vi "poll.vi"(8 "error in (no error)":errorcluster, 11 "output_request_poller in":refnum<class "output_poller.lvclass">) -> (0 "error out":errorcluster, 3 "output_request_poller out":refnum<class "output_poller.lvclass">)   [LabVIEW 2015, in "output_poller.lvclass"]
uses:
  output_poller.lvclass
  output_poller.lvclass/output_poller.ctl
  <vilib>/ActorFramework/Actor/Actor.lvclass/Actor.ctl
  <vilib>/ActorFramework/Message Enqueuer/Message Enqueuer.lvclass/Message Enqueuer.ctl
  <vilib>/ActorFramework/Message Enqueuer/Init from Existing Queue.vi
  <vilib>/ActorFramework/Message Enqueuer/Enqueue.vi
  <vilib>/ActorFramework/Message Priority Queue/Priority Enqueue.vi
  <vilib>/ActorFramework/Stop Msg/Stop Msg.lvclass
  <vilib>/ActorFramework/Message Enqueuer/Message Enqueuer.lvclass
  <vilib>/ActorFramework/Actor/Actor.lvclass
  request/request.lvclass
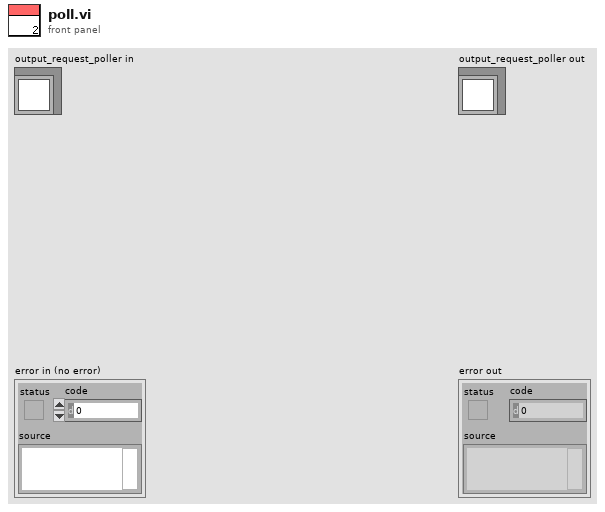
[diagram p1: front panel]
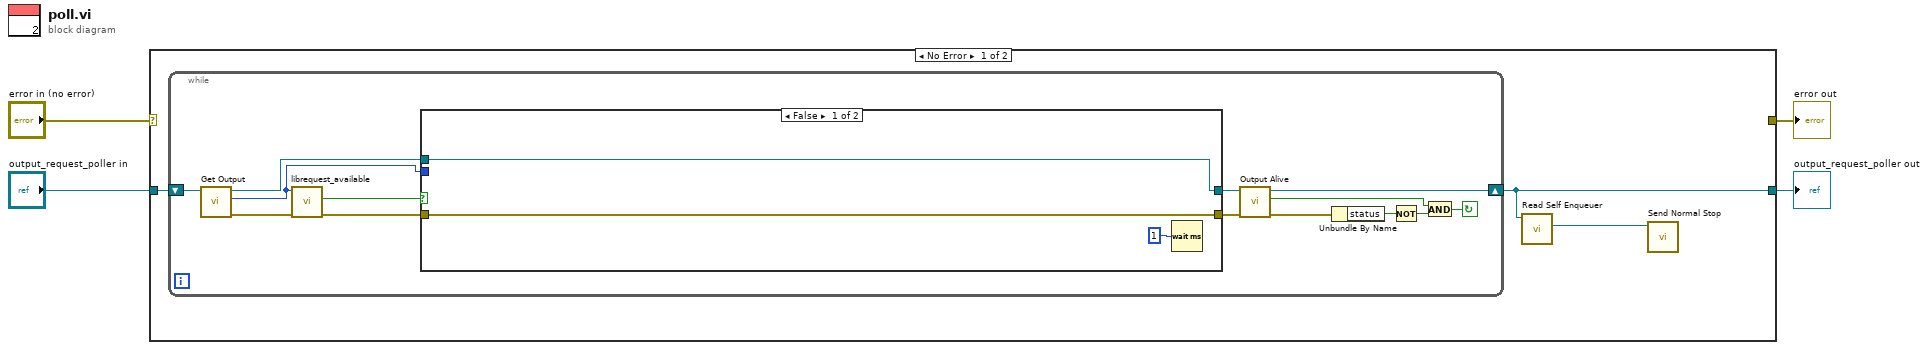
[diagram p0: block diagram]
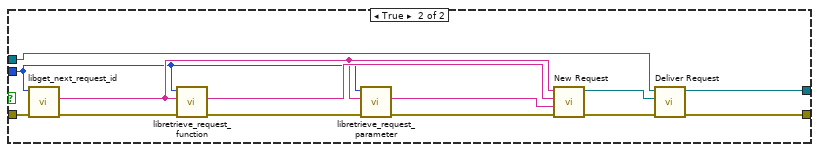
[diagram p2: hidden frame]
diagram:
  n1 = case shown="No Error" "error in (no error)" {
    selector: "error in (no error)" -> [_ w39]
    tunnel: [_ w39] -> w3
    tunnel: [w6 w38] -> w1
    tunnel: "output_request_poller in" -> [w7 w38]
    frame No Error {
      n2 = while {
        shift-right: [w20] -> w6
        shift-left: w7 -> [w17]
        stop <- w8 continue-if-true
        n3 = call "Get Output.vi"("output_request_poller in"=w17) -> ("error out"=w16:errorcluster, "output"=w14:i32, "output_request_poller out"=w15:refnum<class "output_poller.lvclass">)  [unwired: 8 in]
        n4 = call "librequest_available.vi"("error in (no error)"=w16, "output"=w14) -> ("error out"=w18:errorcluster, "is"=w19:bool)  [unwired: 8 in]
        n5 = case shown="False" w19 {
          tunnel: w18 -> [w24 w37]
          tunnel: [w24 w26] -> w21
          tunnel: w15 -> [w22 w29]
          tunnel: w14 -> [_ w30]
          tunnel: [w22 w25] -> w13
          frame False {
            n6 = Wait (ms)(milliseconds to wait=u32 1) -> ()  [unwired: 1 out]
          }
          frame True {
            n7 = call "libget_next_request_id.vi"("error in (no error)"=w37, "output"=w30) -> ("error out"=w36:errorcluster, "id"=w31:string)  [unwired: 8 in]
            n8 = call "libretrieve_request_function.vi"("error in (no error)"=w36, "id"=w31, "output"=w30) -> ("error out"=w35:errorcluster, "function"=w33:string)  [unwired: 7 in]
            n9 = call "libretrieve_request_parameter.vi"("error in (no error)"=w35, "id"=w31, "output"=w30) -> ("error out"=w32:errorcluster, "parameter"=w34:string)  [unwired: 7 in]
            n10 = call "New Request.vi"("error in (no error)"=w32, "params"=w34, "function"=w33, "id"=w31) -> ("error out"=w28:errorcluster, "request"=w27:refnum<class "request.lvclass">)  [unwired: 6 in]
            n11 = call-dynamic "Deliver Request.vi"("error in (no error)"=w28, "Request"=w27, "output_poller in"=w29) -> ("error out"=w26:errorcluster, "output_poller out"=w25:refnum<class "output_poller.lvclass">)  [unwired: 7 in]
          }
        }
        n12 = call "Output Alive.vi"("error in (no error)"=w21, "output_request_poller in"=w13) -> ("error out"=w12:errorcluster, "alive"=w9:bool, "output_request_poller out"=w20:refnum<class "output_poller.lvclass">)  [unwired: 7 in]
        n13 = Unbundle By Name(w12) -> ("status"=w11:bool)
        n14 = Not(x=w11) -> (.not. x?=w10:bool)
        n15 = And(x=w9, y=w10) -> (x .and. y?=w8:bool)
      }
      n16 = call <vilib>:"Read Self Enqueuer.vi"("Actor"=w6) -> ("Self Enqueuer"=w5:refnum<class "Message Enqueuer.lvclass">)  [unwired: 10 in]
      n17 = call <vilib>:"Send Normal Stop.vi"("Message Enqueuer"=w5) -> ()  [unwired: 10 in, 1 out]
    }
    frame Error {
    }
  }
  "error out" <- w3
  "output_request_poller out" <- w1
